vi "PinsToAngle.vi"(6 "Number of pins":i32=8, 7 "Templates path":path=path "C:/Users/Aerotech/Documents/BNL_ThermomechanicalStave/Utils/ConfigurationFiles_and_Templates/0_Calibration", 8 "Sample Size per pin":i32=5, 9 "Pixel to Micron":dbl=1.7483, 10 "Input Image Array":T4[](array[typedef])=["image_000_-644_132_22", "image_001_-644_132_22", "image_002_-644_132_22", "image_003_-632_132_22", "image_004_-632_132_22", "image_005_-632_132_22", "image_006_-364_132_22", "image_007_-364_132_22", "image_008_-364_132_22", "image_009_-352_132_22", "image_010_-352_132_22", "image_011_-352_132_22", "image_012_-70_132_22", "image_013_-70_132_22", "image_014_-70_132_22", "image_015_-58_132_22", "image_016_-58_132_22", "image_017_-58_132_22", "image_018_224_132_22", "image_019_224_132_22", "image_020_224_132_22", "image_021_236_132_22", "image_022_236_132_22", "image_023_236_132_22"], 11 "Input Coordinate Array":dbl[][](array[numeric])=[[-643.9998658385741, 131.9999453490967, 21.9298615361691], [-643.9999903502929, 132.0000069946045, 21.9298615361691], [-644.0000059905517, 131.99999661862793, 21.9298615361691], [-632.000386279907, 132.000063452124, 21.9297615361691], [-631.9999895513914, 132.00000226437987, 21.9298615361691], [-631.999998782959, 131.9999997466797, 21.9298615361691], [-363.95049043534175, 132.00022206723634, 21.9297615361691], [-363.95000162003413, 131.9999977630371, 21.9298615361691], [-363.9500002467431, 132.00000455319824, 21.9298615361691], [-351.95049463707517, 132.0000499480957, 21.9298615361691], [-351.9500095601709, 131.9999912017578, 21.9298615361691], [-351.94999659020016, 131.9999960845703, 21.9298615361691], [-69.94956743774902, 132.00000539243163, 21.9299615361691], [-69.94999994812498, 132.00000516354982, 21.9298615361691], [-69.94999193726075, 132.00000874936524, 21.9298615361691], [-57.9495269084082, 132.00002728879394, 21.9299615361691], [-57.94999748946289, 132.00000577390136, 21.9298615361691], [-57.94999405623535, 131.99999921262207, 21.9298615361691], [224.04980007456544, 131.9999989074463, 21.9298615361691], [224.05000225352052, 131.99999837338868, 21.9298615361691], [224.04999698923828, 131.99998464047852, 21.9298615361691], [236.0496491630761, 132.00008809506835, 21.9297615361691], [236.04999805528803, 131.9999973815674, 21.9298615361691], [236.0499969108789, 131.99999684750978, 21.9298615361691]]) -> (0 "Each point on located edges":T1(graph)=[{"Top averages"=[-619.173082641082, -633.6974050174084, nan, -344.21244291666903, -353.04973055600044, nan, -49.946978057486696, -58.86453188187489, nan, 244.3912465671938, 235.43114147633693, nan, -626.4352438292452, -626.4352438292452, -626.4352438292452, -348.63108673633474, -348.63108673633474, -348.63108673633474, -54.40575496968079, -54.40575496968079, -54.40575496968079, 239.91119402176537, 239.91119402176537, 239.91119402176537], "Best Linear Fit"=[138.84543815864208, 138.84543815864208, 138.84543815864208, 138.2347031742008, 138.2347031742008, 138.2347031742008, 138.6858989969535, 138.6858989969535, 138.6858989969535, 138.1609433697574, 138.1609433697574, 138.1609433697574, 141.04139674590095, 136.6494795713832, nan, 141.0417518521113, 135.4276544962903, nan, 140.3753479525577, 136.99645004134933, nan, 139.8807977818968, 136.441088957618, nan]}, {"Top averages"=[-700.0, -300.0, 100.0, 500.0, 700.0], "Best Linear Fit"=[138.7576137676204, 138.5380654378511, 138.3185171080818, 138.0989687783125, 137.98919461342786]}], 1 "Angle (rad)":dbl=-0.0005488707693057858, 2 "Mean (x,y) T.P stage reference system":dbl[][](array[numeric]), 3 "Average Positions":dbl[][](array[numeric])=[[-626.4352438292452, -348.63108673633474, -54.40575496968079, 239.91119402176537], [138.84543815864208, 138.2347031742008, 138.6858989969535, 138.1609433697574]])   [LabVIEW 2016]
uses:
  <vilib>/vision/Image Controls.llb/IMAQ Image.ctl
  <vilib>/Analysis/6fits.llb/Curve Fitting Criteria.ctl
  <vilib>/Utility/file.llb/Read Delimited Spreadsheet (DBL).vi
  <vilib>/vision/NI_Vision_Development_Module.lvlib
  <vilib>/Analysis/NI_AALPro.lvlib
panel:
  out "Angle (mrad)":dbl
  out "Intercept (mm)":dbl
  in  "x values for fit line on plot":dbl[](array[numeric])=[-700.0, -300.0, 100.0, 500.0, 700.0]
  out "Residue":dbl=0.05294465773658885
  in  "Fit Method":T2 items=["Least Square", "Least Absolute Residual", "Bisquare"]
  out "Position errors":dbl[][](array[numeric])
  in  "Tab Control":T3(tab)
  in  "?":path=path "D:/Iria/ATLAS17/6-10"
  in  "Image file format":string="*.png"
  out "Image File Names":string[](array[string])
  out "Tooling Pin Coordinates":dbl[][](array[numeric])
  in  "Camera coordinate file path":path=path "D:/Iria/ATLAS17/6-10-Coords.csv"
  out "Template Image Right":T4
  out "Template Image Left":T4
  in  "Testing?":bool
  out "Template Left":T4(plugin-control)
  out "Template Right":T4(plugin-control)
  out "Match or no-match?":i32[](array[numeric])
  out "Image Array":T4[](array[plugin-control])
  out "processing image:":i32
  in  "Settings":T5={"Algorithm"=2, "Number of Matches Requested"=1, "Minimum Match Score"=800.0, "SubPixel Accuracy"=TRUE, "Rotation Angle Ranges"=[], "Show Search Area"=FALSE, "Show Result"=TRUE} {"Rotation Angle Ranges"."End" format="%.1f"; "Rotation Angle Ranges"."Start" format="%.1f"; "Minimum Match Score" min=0 max=1000 format="%.2f"; "Number of Matches Requested" min=1; "Algorithm" items=["All", "Low Discrepancy Sampling", "Grayscale Value Pyramid", "Gradients Pyramid"]}
  out "Patterns (mm)":dbl[][](array[numeric])
  # "Pictures directory path"
  # "INPUT NO TESTING"
  # "TESTING"
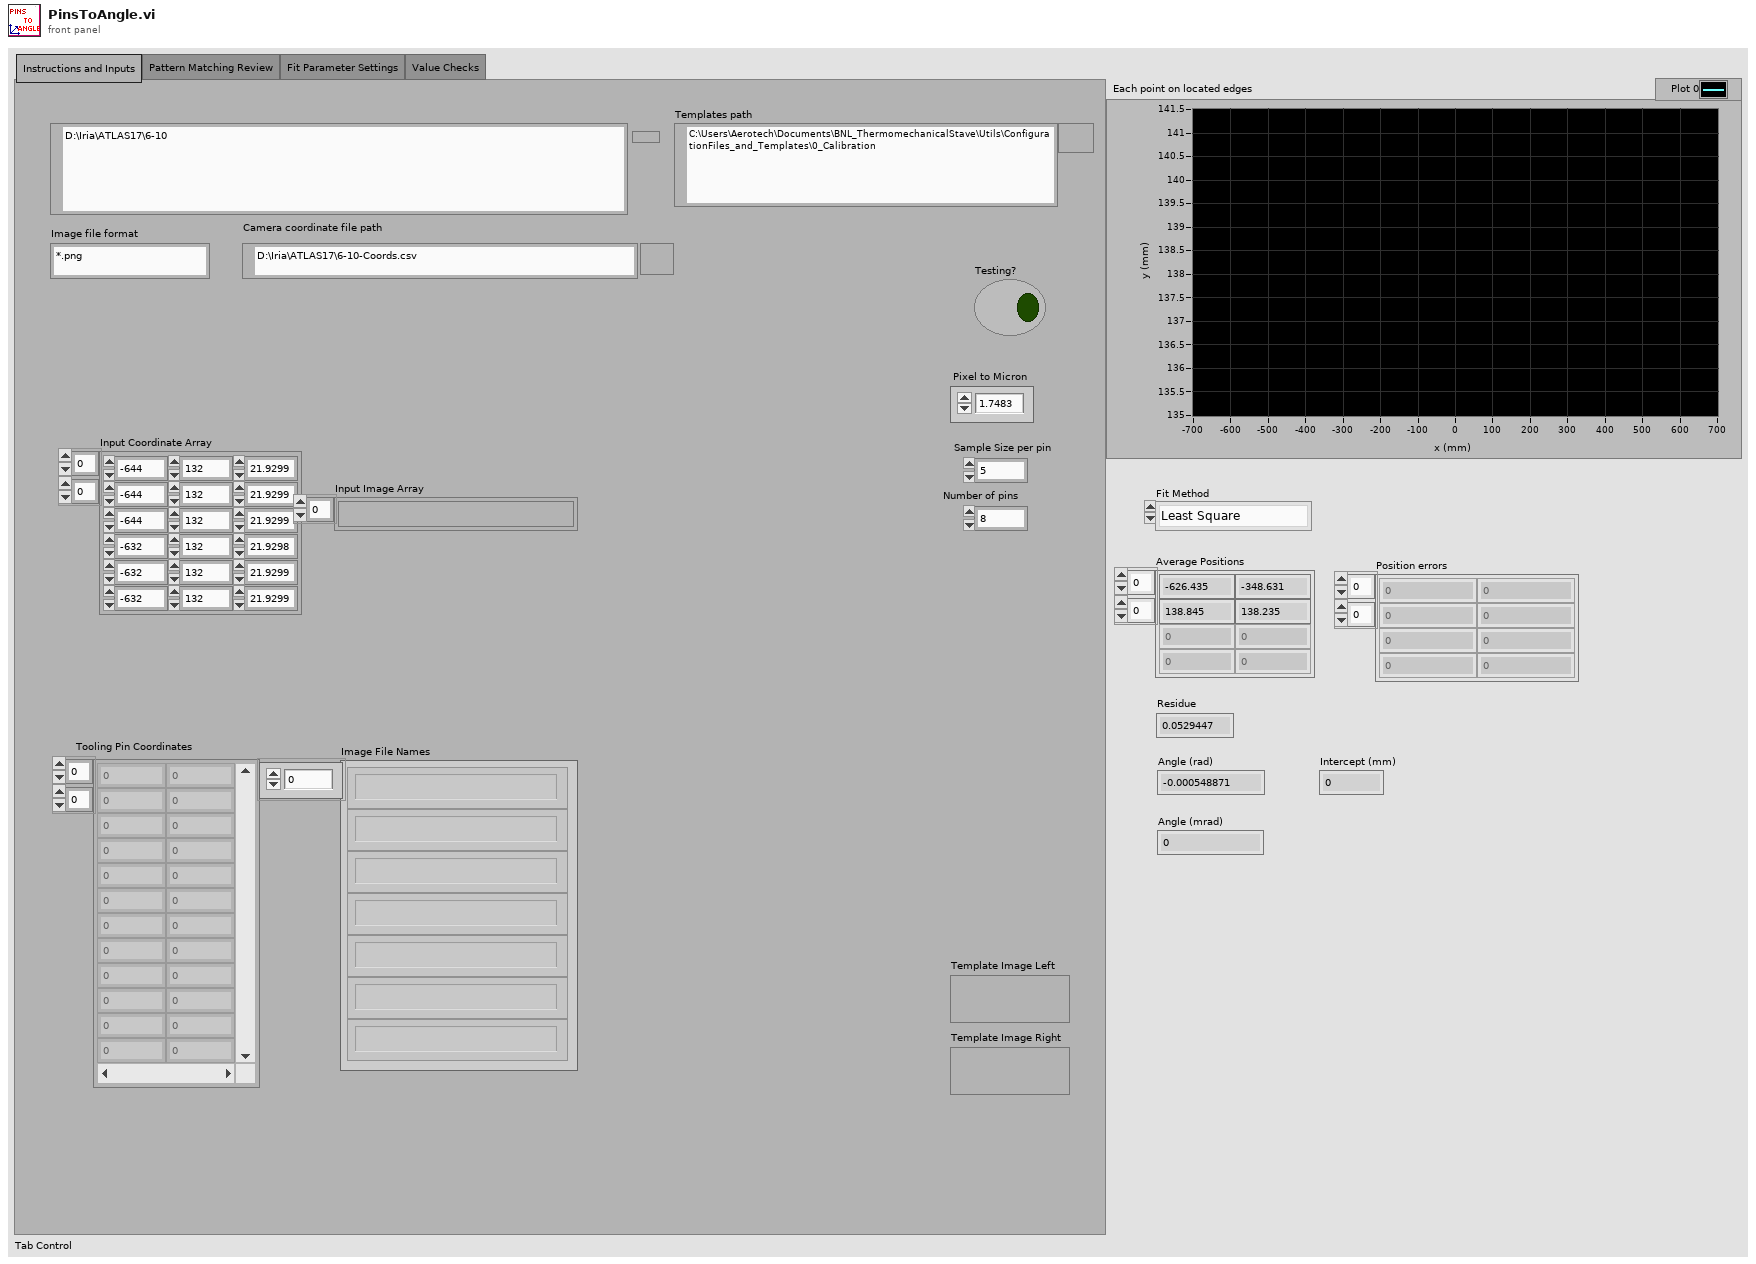
[diagram p1: front panel]
types:
  T1 = cluster{"Top averages":dbl[], "Best Linear Fit":dbl[]}[]
  T2 = typedef "NI_AALPro.lvlib/Curve Fitting Criteria.ctl" = u16
  T3 = enum32{"Instructions and Inputs", "Pattern Matching Review", "Fit Parameter Settings", "Value Checks"}
  T4 = typedef "IMAQ Image.ctl" = refnum<image>
  T5 = cluster{"Algorithm":i32, "Number of Matches Requested":i32, "Minimum Match Score":sgl, "SubPixel Accuracy":bool, "Rotation Angle Ranges":cluster{"Start":sgl, "End":sgl}[], "Show Search Area":bool, "Show Result":bool}
  T6 = typedef "Image Type" = u32
  T7 = cluster{"all rows[0]":dbl, "all rows[1]":dbl, "all rows[2]":dbl, "all rows[3]":dbl, "all rows[4]":dbl, "all rows[5]":dbl, "all rows[6]":dbl, "all rows[7]":dbl, "all rows[8]":dbl}
  T8 = cluster{"Position":cluster{"x":sgl, "y":sgl}, "Angle":sgl, "Scale":sgl, "Score":sgl, "Bounding Box":cluster{"x":sgl, "y":sgl}[]}[]
  T9 = cluster{"Matches (pixel)[0]":cluster{"Position":cluster{"x":sgl, "y":sgl}, "Angle":sgl, "Scale":sgl, "Score":sgl, "Bounding Box":cluster{"x":sgl, "y":sgl}[]}, "Matches (pixel)[1]":cluster{"Position":cluster{"x":sgl, "y":sgl}, "Angle":sgl, "Scale":sgl, "Score":sgl, "Bounding Box":cluster{"x":sgl, "y":sgl}[]}, "Matches (pixel)[2]":cluster{"Position":cluster{"x":sgl, "y":sgl}, "Angle":sgl, "Scale":sgl, "Score":sgl, "Bounding Box":cluster{"x":sgl, "y":sgl}[]}, "Matches (pixel)[3]":cluster{"Position":cluster{"x":sgl, "y":sgl}, "Angle":sgl, "Scale":sgl, "Score":sgl, "Bounding Box":cluster{"x":sgl, "y":sgl}[]}, "Matches (pixel)[4]":cluster{"Position":cluster{"x":sgl, "y":sgl}, "Angle":sgl, "Scale":sgl, "Score":sgl, "Bounding Box":cluster{"x":sgl, "y":sgl}[]}, "Matches (pixel)[5]":cluster{"Position":cluster{"x":sgl, "y":sgl}, "Angle":sgl, "Scale":sgl, "Score":sgl, "Bounding Box":cluster{"x":sgl, "y":sgl}[]}, "Matches (pixel)[6]":cluster{"Position":cluster{"x":sgl, "y":sgl}, "Angle":sgl, "Scale":sgl, "Score":sgl, "Bounding Box":cluster{"x":sgl, "y":sgl}[]}, "Matches (pixel)[7]":cluster{"Position":cluster{"x":sgl, "y":sgl}, "Angle":sgl, "Scale":sgl, "Score":sgl, "Bounding Box":cluster{"x":sgl, "y":sgl}[]}, "Matches (pixel)[8]":cluster{"Position":cluster{"x":sgl, "y":sgl}, "Angle":sgl, "Scale":sgl, "Score":sgl, "Bounding Box":cluster{"x":sgl, "y":sgl}[]}}
  T10 = cluster{"Position":cluster{"x":sgl, "y":sgl}, "Angle":sgl, "Scale":sgl, "Score":sgl, "Bounding Box":cluster{"x":sgl, "y":sgl}[]}
  T11 = cluster{"x values for fit line on plot":dbl[], "Array":dbl[]}
  T12 = cluster{"x values for fit line on plot":dbl[], "Array":dbl[]}[]
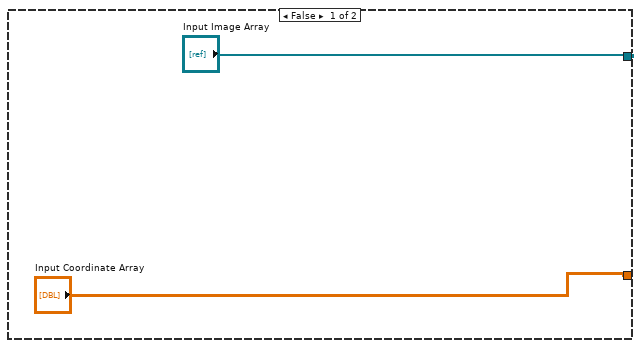
[diagram p2: hidden frame]
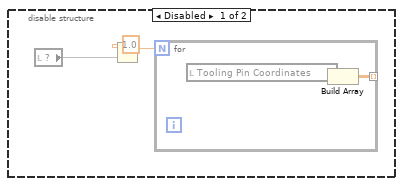
[diagram p4: hidden frame]
diagram:
  n1 = flat-sequence {
    tunnel: [w24] -> w3
    tunnel: [w8] -> w2
    tunnel: [w7] -> w1
    tunnel: w3 -> [w80]
    tunnel: w2 -> [w77]
    tunnel: w1 -> [w76]
    tunnel: [w78] -> _
    frame #0 {
      # "Locking Point\nPattern Template"
      # "Locking Point\nPattern Template"
      n2 = case shown="True" "Testing?" {
        tunnel: ["Input Image Array" w34] -> w24
        tunnel: ["Input Coordinate Array" w32] -> w5
        frame False {
        }
        frame True {
          n3 = List Folder(path="?", pattern="Image file format") -> (path out=w37:path, filenames=w35:string[])  [unwired: 2 in, 2 out]
          "Image File Names" <- w35
          n4 = call-poly <vilib>:"Read Delimited Spreadsheet.vi"("file path (dialog if empty)"="Camera coordinate file path", "format (%.3f)"="%.9f", "delimiter (\\t)"="," ("Delimiter")) -> ("all rows"=w32:dbl[][])  [unwired: 7 in, 5 out]
          "Tooling Pin Coordinates" <- w32
          n5 = for {
            tunnel: w37 -> [w43]
            tunnel: w35 -> [w42] mode=indexing
            tunnel: [w41] -> w34 mode=indexing
            w45 = T6 0 items=["Grayscale (U8)", "Grayscale (I16)", "Grayscale (SGL)", "Complex (CSG)", "RGB (U32)", "HSL (U32)", "RGB (U64)", "Grayscale (U16)"] ("Image Type")
            n6 = Build Path(base path=w43, name or relative path=w42) -> (appended path=w47:path)
            n7 = call "IMAQ Create"("Image Name"=w42, "Image Type"=w45) -> ("New Image"=w44:T4, "error out"=w46:errorcluster)  [unwired: 3 in]
            n8 = call "IMAQ ReadFile"("File Path"=w47, "error in (no error)"=w46, "Image"=w44) -> ("Image Out"=w41:T4)  [unwired: 4 in, 4 out]
          }
        }
      }
      n9 = Build Path(base path="Templates path", name or relative path="2_StaveCoordinateSystem") -> (appended path=w19:path)
      n10 = Build Path(base path=w19, name or relative path="ToolingPin-Right.png") -> (appended path=w11:path)
      n11 = call "IMAQ Create"("Image Name"="rightroi") -> ("New Image"=w22:T4, "error out"=w21:errorcluster)  [unwired: 4 in]
      n12 = Build Path(base path="Templates path", name or relative path="2_StaveCoordinateSystem") -> (appended path=w13:path)
      n13 = call "IMAQ ReadFile"("File Path"=w11, "error in (no error)"=w21, "Image"=w22) -> ("Image Out"=w8:T4)  [unwired: 4 in, 4 out]
      "Template Image Right" <- w8
      "Template Right" <- w8
      n14 = call "IMAQ Create"("Image Name"="leftroi") -> ("New Image"=w16:T4, "error out"=w15:errorcluster)  [unwired: 4 in]
      n15 = Build Path(base path=w13, name or relative path="ToolingPin-Left.png") -> (appended path=w10:path)
      n16 = call "IMAQ ReadFile"("File Path"=w10, "error in (no error)"=w15, "Image"=w16) -> ("Image Out"=w7:T4)  [unwired: 4 in, 4 out]
      "Template Image Left" <- w7
      "Template Left" <- w7
      n17 = for {
        tunnel: w5 -> [w29] mode=indexing
        tunnel: [w28] -> w4 mode=indexing
        n18 = Array To Cluster(array=w29) -> (cluster=w25:T7)
        n19 = Unbundle By Name(w25) -> ("all rows[0]"=w27:dbl, "all rows[1]"=w26:dbl)
        n20 = Build Array(w27, w26) -> (w28:dbl[])
      }
      n21 = local write "Tooling Pin Coordinates"(w4) -> ()
    }
    frame #1 {
      # "Next we average points for each of the pictures. and calculate errors on them"
      n22 = for {
        tunnel: w80 -> [w88] mode=indexing
        tunnel: [w89] -> w78 mode=indexing
        tunnel: [w87] -> w79 mode=indexing
        tunnel: w77 -> [w85]
        tunnel: w76 -> [w84]
        tunnel: [w83] -> _ mode=indexing
        tunnel: [w82] -> w48 mode=indexing
        tunnel: ["Sample Size per pin"] -> w49
        i -> [w86]
        n23 = flat-sequence {
          tunnel: w86 -> [w95]
          tunnel: w88 -> [w116]
          tunnel: [w111] -> w89
          tunnel: [w114] -> w87
          tunnel: w85 -> [w105]
          tunnel: w84 -> [w104]
          tunnel: [w99] -> w83
          tunnel: [w98] -> w82
          tunnel: "Sample Size per pin" -> [w97]
          frame #0 {
            w124 = 2 ("y")
            n24 = local read "Tooling Pin Coordinates"() -> (w96:dbl[][])
            n25 = Index Array(array=w96, index (row)=w95) -> (element=w94:dbl[])  [unwired: 1 in]
            n26 = Index Array(array=w94, index #1=0 ("index"), index #2=1 ("index")) -> (element #1=w91:dbl, element #2=w90:dbl)
            n27 = call "IMAQ GetImageSize"("Image"=w116) -> ("Y Resolution"=w123:i32, "X Resolution"=w122:i32)  [unwired: 3 in, 1 out]
            n28 = Divide(x=w122, y=w124) -> (x/y=w125:dbl)
            n29 = Divide(x=w123, y=w124) -> (x/y=w127:dbl)
            n30 = Quotient & Remainder(x=w95, y=w97) -> (floor(x/y)=w108:i32)  [unwired: 1 out]
            n31 = local read "Image Array"() -> (w112:T4[])
            n32 = Quotient & Remainder(x=w108, y=2) -> (x-y*floor(x/y)=w106:i32)  [unwired: 1 out]
            n33 = case shown="1" w106 {
              tunnel: [w132 w133] -> w107
              tunnel: w105 -> [w132 _]
              tunnel: w104 -> [_ w133]
              frame 0, Default {
              }
              frame 1 {
              }
            }
            n34 = call "IMAQ Find Pattern 4"("Image"=w116, "Template"=w107, "Settings"="Settings") -> ("Number of Matches"=w114:i32, "Image Out"=w111:T4, "Matches (pixel)"=w118:T8)  [unwired: 6 in, 4 out]
            n35 = Array To Cluster(array=w118) -> (cluster=w119:T9)
            n36 = Unbundle By Name(w119) -> ("Matches (pixel)[0]"=w120:T10)
            n37 = Replace Array Subset(array=w112, new element=w111, index=w95) -> (w110:T4[])
            n38 = Unbundle By Name(w120) -> ("Position"=w121:cluster{"x":sgl, "y":sgl})
            n39 = local write "Image Array"(w110) -> ()
            n40 = Unbundle By Name(w121) -> ("x"=w126:sgl, "y"=w128:sgl)
            n41 = Subtract(x=w126, y=w125) -> (x-y=w130:dbl)
            n42 = Subtract(x=w128, y=w127) -> (x-y=w131:dbl)
            n43 = Divide(x="Pixel to Micron", y=1000.0) -> (x/y=w129:dbl)
            n44 = Multiply(x=w129, y=w130) -> (x*y=w103:dbl)
            n45 = Multiply(x=w129, y=w131) -> (x*y=w102:dbl)
            n46 = Add(x=w103, y=w91) -> (x+y=w101:dbl)
            n47 = Subtract(x=w90, y=w102) -> (x-y=w100:dbl)
            n48 = Build Array(w103, w102) -> (w99:dbl[])
            n49 = Build Array(w101, w100) -> (w98:dbl[])
            "processing image:" <- w95
          }
        }
      }
      "Match or no-match?" <- w79
      "Patterns (mm)" <- w48
      n50 = local write "Image Array"(w78) -> ()
      n51 = call "Average2DArrayofSamples.vi"("Sample Size"=w49, "Number of Samples"="Number of pins", "2D Array of Samples"=w48) -> ("Std Devs"=w75:dbl[][], "Averages"=w71:dbl[][])
      "Mean (x,y) T.P stage reference system" <- w71
      n52 = call "Findmidpoints-Toolingpinsutility.vi"("2D Array of Error"=w75, "2D Array of Data"=w71, "Sample Size"="Number of pins") -> ("Std Devs"=w72:dbl[][], "Averages"=w73:dbl[][])  [unwired: 7 in]
      "Average Positions" <- w73
      "Position errors" <- w72
      n53 = Index Array(array=w73, index (col)=0 ("disabled index (col)")) -> (element=w64:dbl[])  [unwired: 1 in]
      n54 = Index Array(array=w73, index (col)=1 ("disabled index (col)")) -> (element=w65:dbl[])  [unwired: 1 in]
      n55 = Index Array(array=w72, index (col)=0) -> (element=w63:dbl[])  [unwired: 1 in]
      n56 = Index Array(array=w72, index (row)=1) -> (element=w50:dbl[])  [unwired: 1 in]
      n57 = call <vilib>:"Linear Fit.vi"("Y"=w65, "X"=w64, "method"="Fit Method") -> ("slope"=w55:dbl, "intercept"=w67:dbl, "residue"=→"Residue":dbl)  [unwired: 8 in, 2 out]
      "Intercept (mm)" <- w67
      n58 = Bundle("Averages"=w64, "Averages"=w65) -> (w66:cluster{"\nAverages":dbl[], "\nAverages":dbl[]})  [unwired: 1 in]
      n59 = Inverse Tangent(1:w55) -> (0:w68:dbl)
      "Angle (rad)" <- w68
      n60 = Multiply(x=1000.0, y=w68) -> (x*y=→"Angle (mrad)":dbl)
      n61 = call "CreatePointsOnLine (SubVI).vi"("x values for fit line on plot"="x values for fit line on plot", "intercept"=w67, "slope"=w55) -> ("Array"=w58:dbl[])  [unwired: 8 in]
      n62 = call "XY error bars.vi"("XY plot"=w66, "Xerror"=w63, "Yerror"=w50) -> ("X+Y error bars"=w61:cluster{dbl[], dbl[]})  [unwired: 5 in, 2 out]
      n63 = Bundle("x values for fit line on plot"="x values for fit line on plot", "Array"=w58) -> (w59:T11)  [unwired: 1 in]
      n64 = Build Array(w61, w59) -> (→"Each point on located edges":T12)
      "Image Array" <- w80
    }
  }
  n65 = disable-structure shown="Enabled" {
    frame Disabled {
      n66 = local read item#-1() -> (w137)
      n67 = Subtract(x=1.0, y=w137) -> (x-y=w136:dbl)
      n68 = for {
        N: w136 -> [_]
        tunnel: [w139] -> w134 mode=indexing
        n69 = local read "Tooling Pin Coordinates"() -> (w138:dbl[][])
        n70 = Build Array(w138) -> (w139:dbl[][][])  [unwired: 1 in]
      }
    }
    frame Enabled {
    }
  }
